vi "Close Hardware.vi"(8 "error in (no error)":errorcluster, 11 "Instrument.FrameworkTemplate":refnum<class "Temperhum.PCSensor.lvclass">) -> (0 "error out":errorcluster, 3 "Instrument.FrameworkTemplate out":refnum<class "Temperhum.PCSensor.lvclass">)   [LabVIEW 2019, in "Temperhum.PCSensor.lvclass"]
uses:
  Temperhum.PCSensor.lvclass
  Temperhum.PCSensor.lvclass/Temperhum.PCSensor.ctl
  Instrument.Temperhum/Instrument.Temperhum.lvclass
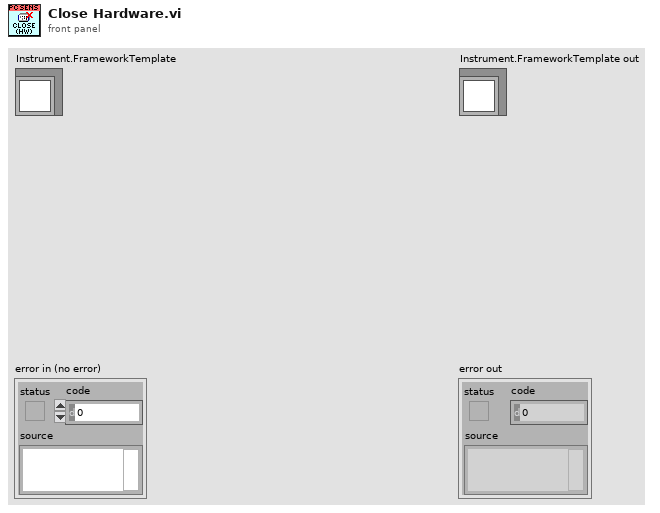
[diagram p1: front panel]
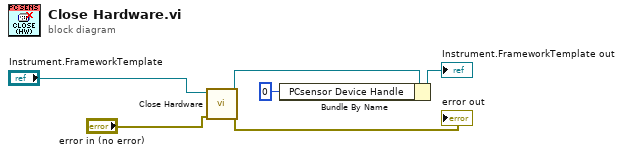
[diagram p0: block diagram]
diagram:
  n1 = call-parent "Close Hardware.vi"("error in (no error)"="error in (no error)", "Instrument.FrameworkTemplate"="Instrument.FrameworkTemplate") -> ("error out"=→"error out":errorcluster, "Instrument.FrameworkTemplate out"=w2:refnum<class "Temperhum.PCSensor.lvclass">)  [unwired: 8 in]
  n2 = Bundle By Name(cluster=w2, "PCsensor Device Handle"=i64 0 ("Device Handle")) -> (→"Instrument.FrameworkTemplate out":refnum<class "Temperhum.PCSensor.lvclass">)
